vi "Do.vi"(8 "error in (no error)":errorcluster, 10 "Actor in":refnum<class "Actor.lvclass">, 11 "Last Ack":refnum<class "Last Ack.lvclass">) -> (0 "error out":errorcluster, 2 "Actor out":refnum<class "Actor.lvclass">)   [LabVIEW 2017, in "Actor Framework.lvlib" / "Last Ack.lvclass"]
uses:
  Last Ack.lvclass
  Actor/Actor.lvclass
  Actor/Actor.lvclass/Actor.ctl
  Read Caller-To-Actor Enqueuer.vi
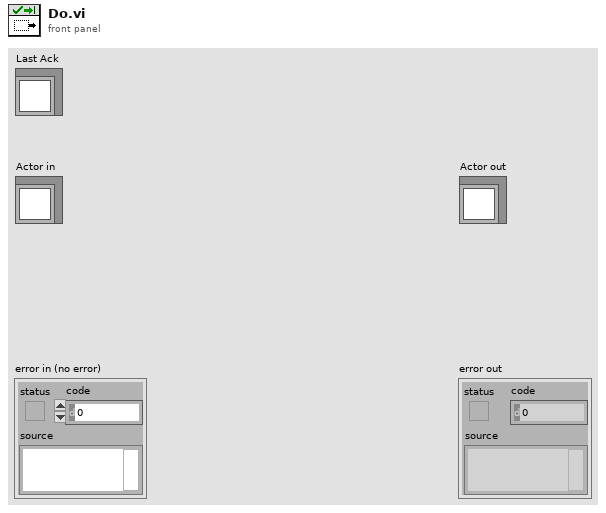
[diagram p1: front panel]
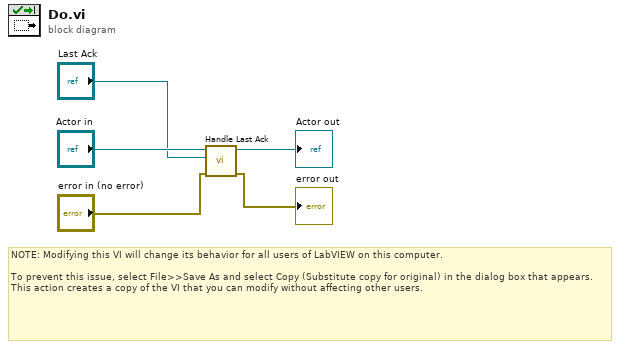
[diagram p0: block diagram]
diagram:
  # "NOTE: Modifying this VI will change its behavior for all users of LabVIEW on this computer.\n\nTo prevent this issue, select File>>Save As and select Copy (Substitute copy for original) in the dialog box that appears. This action creates a copy of the VI that you can modify without affecting other users."
  n1 = call "Handle Last Ack.vi"("error in (no error)"="error in (no error)", "Last Ack"="Last Ack", "Actor in"="Actor in") -> ("error out"=→"error out":errorcluster, "Actor out"=→"Actor out":refnum<class "Actor.lvclass">)  [unwired: 7 in]
